vi "Insert.vi"(6 "Time Stamp":timestamp, 8 "error in":errorcluster, 9 "Data":variant, 10 "Paths (string or array of strings)":variant, 11 "Data.PG in":refnum<class "Data.PG.lvclass">) -> (0 "error out":errorcluster, 3 "Data.PG out":refnum<class "Data.PG.lvclass">)   [LabVIEW 2020, in "Data.PG.lvclass"]
uses:
  Data.PG.lvclass
  <vilib>/JDP Science/PostgreSQL Library/Connection/PQ Connection.lvclass
  Data/Typedefs/Operation--enum.ctl
  Data/Data.lvclass
  <vilib>/JDP Science/PostgreSQL Library/Connection/Execute Command (No results).vi
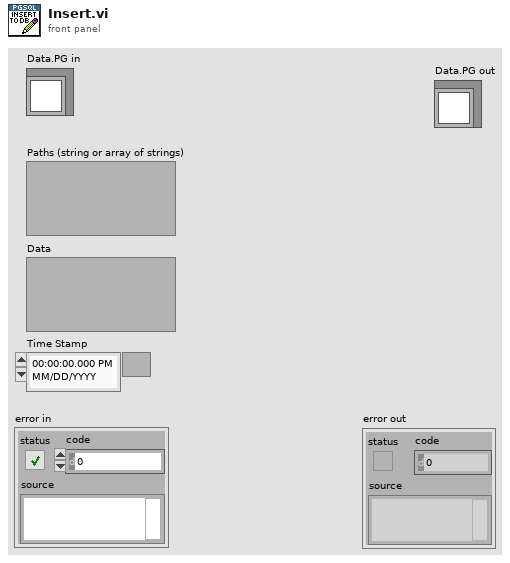
[diagram p1: front panel]
types:
  T1 = typedef "Data.lvclass/Operation--enum.ctl" = enum16{"Read", "Write", "Write + Append"}
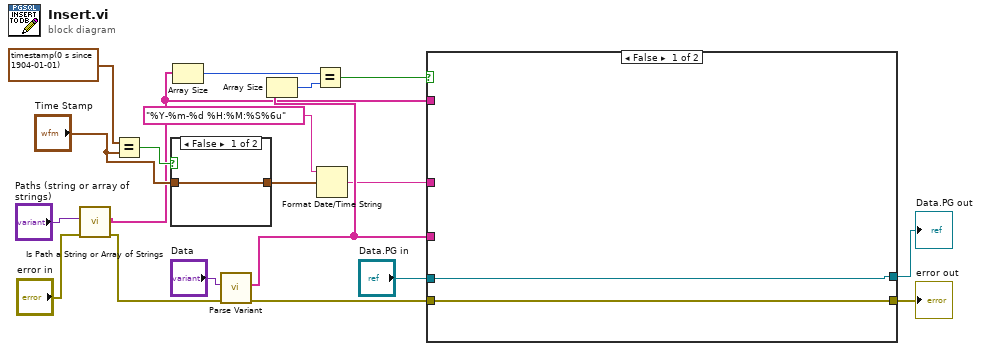
[diagram p0: block diagram]
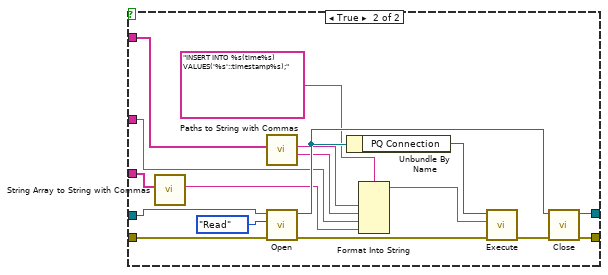
[diagram p2: hidden frame]
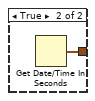
[diagram p3: hidden frame]
diagram:
  n1 = call "Is Path a String or Array of Strings.vi"("error in"="error in", "Paths?"="Paths (string or array of strings)") -> ("error out"=w1:errorcluster, "Paths."=w3:string[])  [unwired: 8 in]
  n2 = Equal?(x=timestamp(0 s since 1904-01-01), y="Time Stamp") -> (x = y?=w16:bool)
  n3 = case shown="False" w16 {
    tunnel: [w20 w21] -> w17
    tunnel: "Time Stamp" -> [w20 _]
    frame False {
    }
    frame True {
      n4 = Get Date/Time In Seconds() -> (seconds since 1Jan1904=w21:timestamp)
    }
  }
  n5 = Array Size(array=w3) -> (size(s)=w13:i32)
  n6 = call "Parse Variant.vi"("error in"=w1, "variant"="Data") -> ("error out"=w8:errorcluster, "Strings"=w10:string[])  [unwired: 6 in, 2 out]
  n7 = Array Size(array=w10) -> (size(s)=w12:i32)
  n8 = Equal?(x=w13, y=w12) -> (x = y?=w11:bool)
  n9 = Format Date/Time String(time format string (%c)="%Y-%m-%d %H:%M:%S%6u", seconds (now)=w17) -> (date/time string=w7:string)  [unwired: 1 in]
  n10 = case shown="False" w11 {
    tunnel: w10 -> [_ w40]
    tunnel: w3 -> [_ w39]
    tunnel: [w23 w34] -> w9
    tunnel: w8 -> [w23 w33]
    tunnel: w7 -> [_ w28]
    tunnel: "Data.PG in" -> [w22 w26]
    tunnel: [w22 w24] -> w5
    frame False {
    }
    frame True {
      n11 = call "String Array to String with Commas.vi"("Array"=w40) -> ("String"=w27:string)  [unwired: 10 in]
      n12 = call "Paths to String with Commas.vi"("Array"=w39) -> ("Columns"=w29:string, "Table"=w30:string)  [unwired: 9 in]
      n13 = call-dynamic "Open.vi"("error in (no error)"=w33, "Operation"=Operation--enum."Read", "Data.PG in"=w26) -> ("error out"=w37:errorcluster, "Data.PG out"=w35:refnum<class "Data.PG.lvclass">)  [unwired: 7 in]
      n14 = Unbundle By Name(w35) -> ("PQ Connection"=w25:refnum<class "PQ Connection.lvclass">)
      n15 = Format Into String(format string="INSERT INTO %s(time%s) VALUES('%s'::timestamp%s);", w30, w29, w28, w27) -> (resulting string=w31:string)  [unwired: 2 in, 1 out]
      n16 = call-poly <vilib>:"Execute.vi"("error in (no error)"=w37, "SQL"=w31, "PQ Connection in"=w25) -> ("error out"=w36:errorcluster)  [unwired: 7 in, 1 out]
      n17 = call-dynamic "Close.vi"("error in (no error)"=w36, "Data.PG in"=w35) -> ("error out"=w34:errorcluster, "Data.PG out"=w24:refnum<class "Data.PG.lvclass">)  [unwired: 8 in]
    }
  }
  "error out" <- w9
  "Data.PG out" <- w5
